vi "Initialize MeasurementLink Session.vi"(7 "remote connection options":T2, 8 "error in":errorcluster, 9 "initialize and close session behavior":T1, 10 "session initialization parameters":T3, 11 "session factory in":refnum<class "Session Factory.lvclass">) -> (0 "error out":errorcluster, 2 "session out":variant, 3 "session factory out":refnum<class "Session Factory.lvclass">)   [LabVIEW 2020, in "Plug-In SDK niDCPower Sessions.lvlib" / "Session Factory.lvclass"]
uses:
  Session Factory.lvclass
  <instrlib>/niDCPower/nidcpower.llb/niDCPower Initialize With Independent Channels for gRPC session.vi
  <instrlib>/niDCPower/nidcpower.llb/niDCPower Attach gRPC session.vi
  Instrument Sessions/ISession Factory/ISession Factory.lvclass
  Instrument Sessions/ISession Factory/Remote Connection Options.ctl
  Instrument Sessions/ISession Factory/Initialize and Close Session Behavior.ctl
  Instrument Sessions/ISession Factory/Session Initialization Parameters.ctl
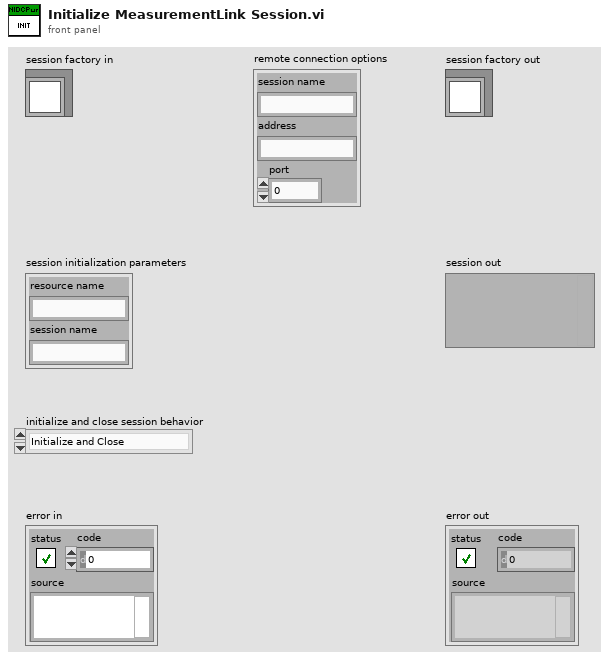
[diagram p1: front panel]
types:
  T1 = typedef "Plug-In SDK Instrument Sessions.lvlib/ISession Factory.lvclass/Initialize and Close Session Behavior.ctl" = enum16{"Initialize and Close", "Attach and Detach", "Initialize and Detach", "Attach and Close"}
  T2 = typedef "Plug-In SDK Instrument Sessions.lvlib/ISession Factory.lvclass/Remote Connection Options.ctl" = cluster{"session name":string, "address":string, "port":u32}
  T3 = typedef "Plug-In SDK Instrument Sessions.lvlib/ISession Factory.lvclass/Session Initialization Parameters.ctl" = cluster{"resource name":string, "session name":string}
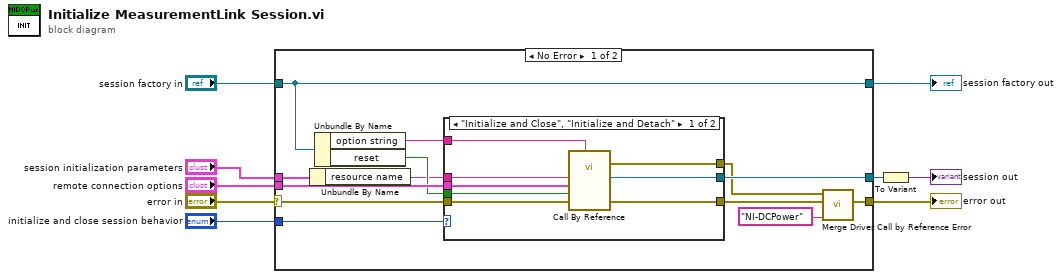
[diagram p0: block diagram]
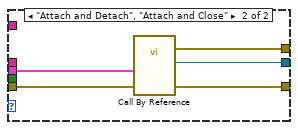
[diagram p2: hidden frame]
diagram:
  n1 = case shown="No Error" "error in" {
    selector: "error in" -> [w19 w36]
    tunnel: [w11 w36] -> w8
    tunnel: "session factory in" -> [w17 w37]
    tunnel: [w17 w37] -> w6
    tunnel: "initialize and close session behavior" -> [w22 _]
    tunnel: "remote connection options" -> [w21 _]
    tunnel: "session initialization parameters" -> [w18 _]
    tunnel: [w20 _] -> w2
    frame No Error {
      n2 = Unbundle By Name(w18) -> ("resource name"=w14:string)
      n3 = Unbundle By Name(w17) -> ("option string"=w16:string, "reset"=w15:bool)
      n4 = case shown="\"Initialize and Close\", \"Initialize and Detach\"" w22 {
        tunnel: w21 -> [w29 w35]
        tunnel: [w28 w34] -> w20
        tunnel: w19 -> [w30 w33]
        tunnel: [w24 w32] -> w13
        tunnel: w14 -> [w27 _]
        tunnel: w16 -> [w26 _]
        tunnel: w15 -> [w25 _]
        tunnel: [w23 w31] -> w12
        frame "Initialize and Close", "Initialize and Detach" {
          n5 = call-by-ref "?"("option string"=w26, "error in (no error)"=w30, "reset (false)"=w25, "gRPC options"=w29, "resource name"=w27) -> (error out=w23:errorcluster, 0:"error out"=w24:errorcluster, "instrument handle out"=w28:refnum<k15>)  [unwired: 7 in, 1 out]
        }
        frame "Attach and Detach", "Attach and Close" {
          n6 = call-by-ref "?"("error in (no error)"=w33, "gRPC options"=w35) -> (error out=w31:errorcluster, 0:"error out"=w32:errorcluster, "instrument handle out"=w34:refnum<k15>)  [unwired: 10 in, 1 out]
        }
      }
      n7 = call "Merge Driver Call by Reference Error.vi"("driver name"="NI-DCPower", "called vi error"=w13, "call by ref error"=w12) -> ("error out"=w11:errorcluster)  [unwired: 8 in]
    }
    frame Error {
    }
  }
  "error out" <- w8
  "session factory out" <- w6
  n8 = To Variant(anything=w2) -> (Variant=→"session out":variant)
